vi "create instrument.vi"() -> ()   [LabVIEW 2020, in "Data.PG.lvclass"]
uses:
  Data.PG.lvclass
  <vilib>/numeric/Random Number (Range) U64.vi
  <vilib>/numeric/sub_Random U32.vi
  <vilib>/ErrorRing/Error Ring.xnode
panel:
  in  "Delete instrument":bool
  in  "Users":i32(listbox)
  out "new password":string
  out "new user name":string
  in  "path to object in table":string
  in  "new instrument password":string
  in  "Create instrument":bool
  in  "generate random password?":bool
  in  "new instrument name":string
  in  "STOP":bool
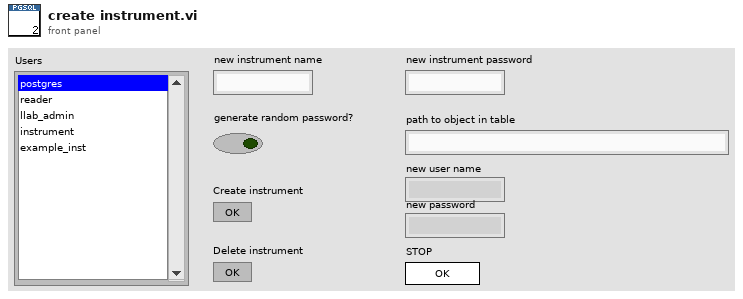
[diagram p1: front panel]
types:
  T1 = enum32{"Invalid", "Standard", "Closed", "Hidden", "Minimized", "Maximized"}
  T2 = enum32{"invalid app kind", "Development System", "Run Time System", "Student Edition", "Embedded LabVIEW", "Evaluation", "Custom"}
  T3 = cluster{"Core":cluster{"Current VI Reference":refnum<vi>, "Close Panel on Exit?":bool}, "connection info":cluster{"host":string, "port":string, "dbname":string, "user":string, "password":string}, "path to something in table":string, "new instrument name":string, "names already taken":string[], "Data.PG in":refnum<class "Data.PG.lvclass">, "Selected instrument":string, "Selected inst privileges":string[]}
  T4 = cluster{"host":string, "port":string, "dbname":string, "user":string, "password":string}
  T5 = cluster{"Current VI Reference":refnum<vi>, "Close Panel on Exit?":bool}
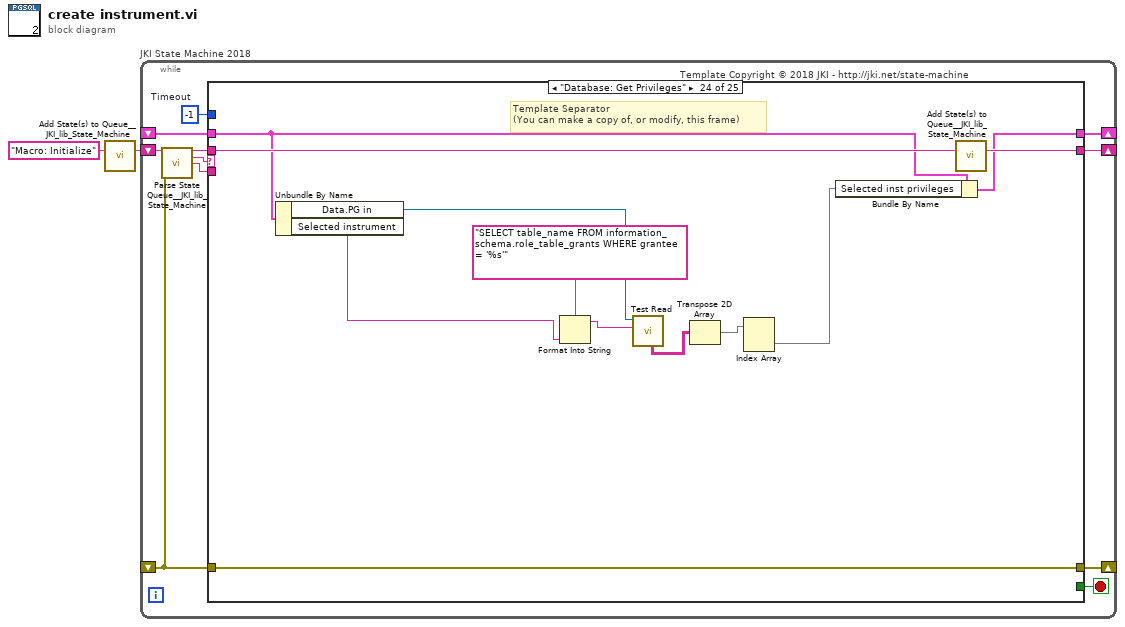
[diagram p0: block diagram]
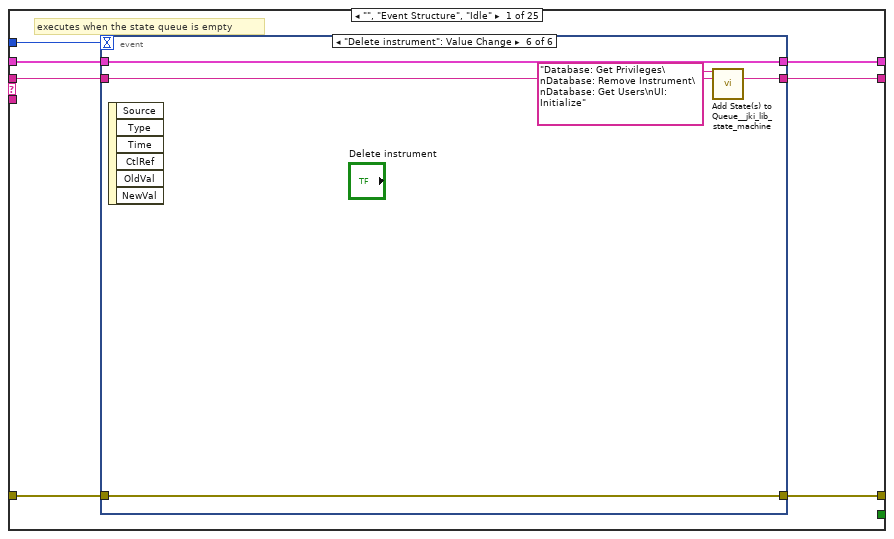
[diagram p2: hidden frame]
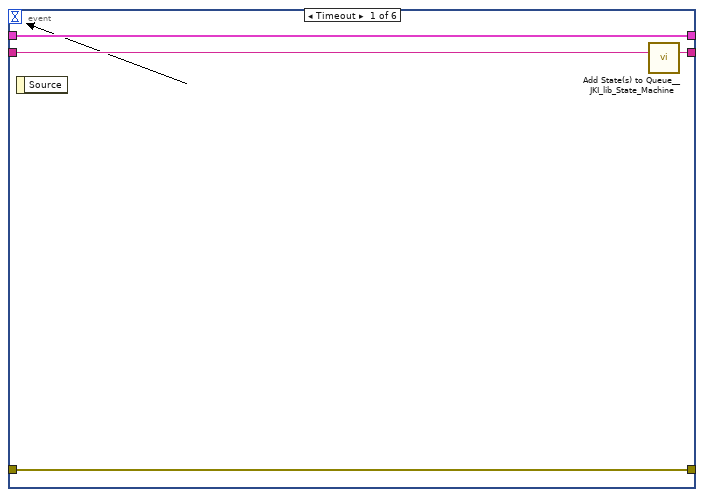
[diagram p3: hidden frame]
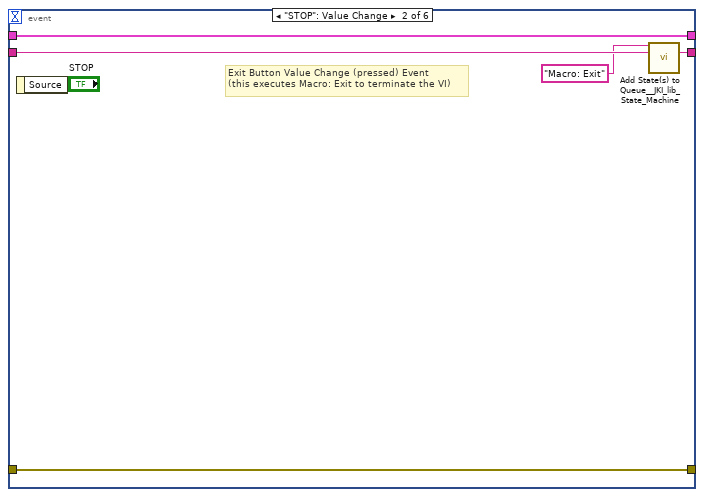
[diagram p4: hidden frame]
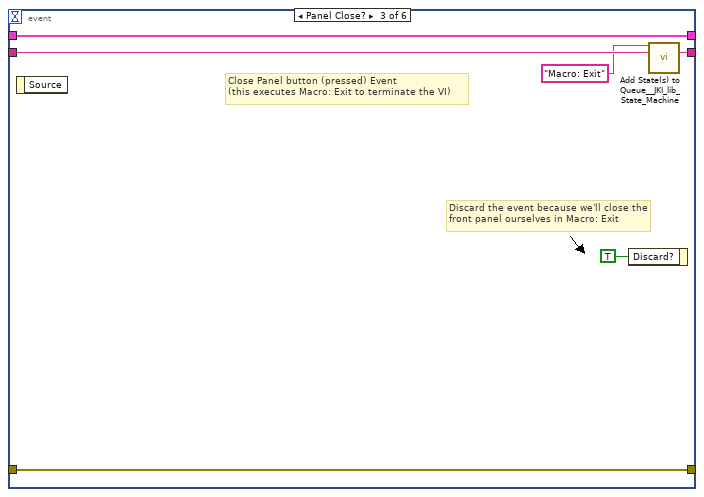
[diagram p5: hidden frame]
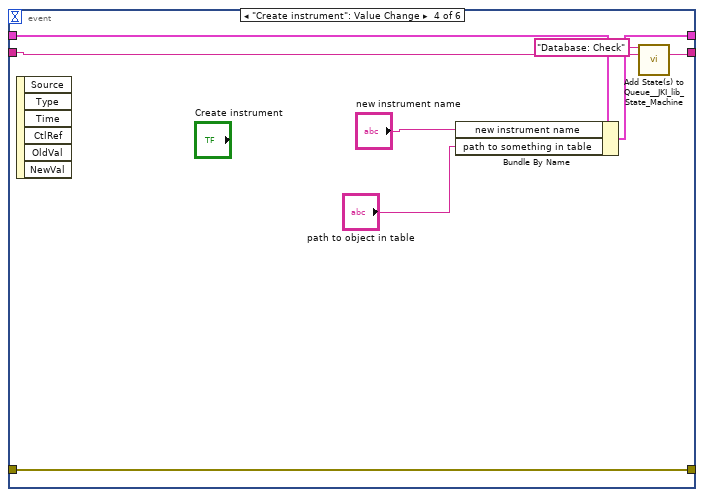
[diagram p6: hidden frame]
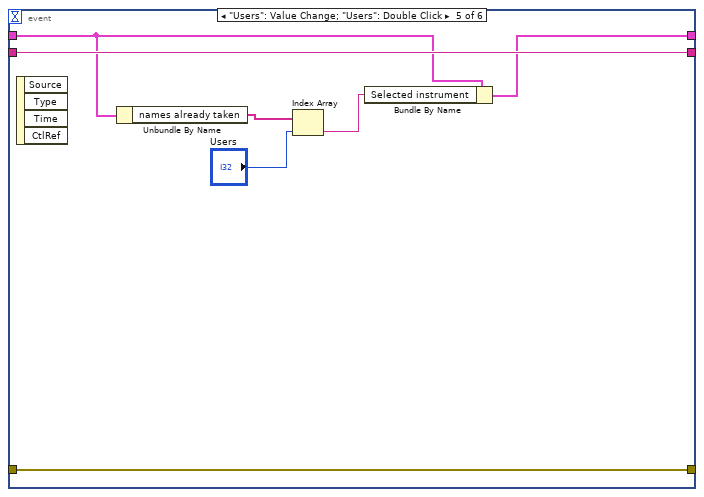
[diagram p7: hidden frame]
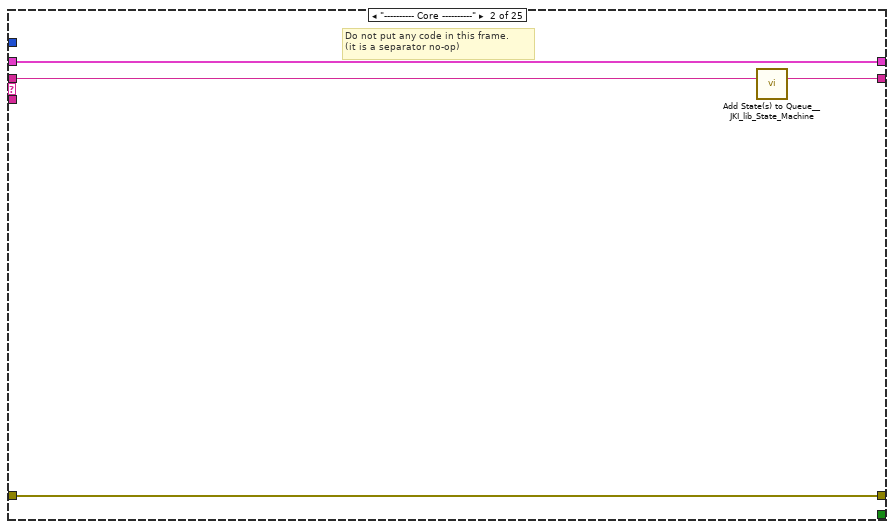
[diagram p8: hidden frame]
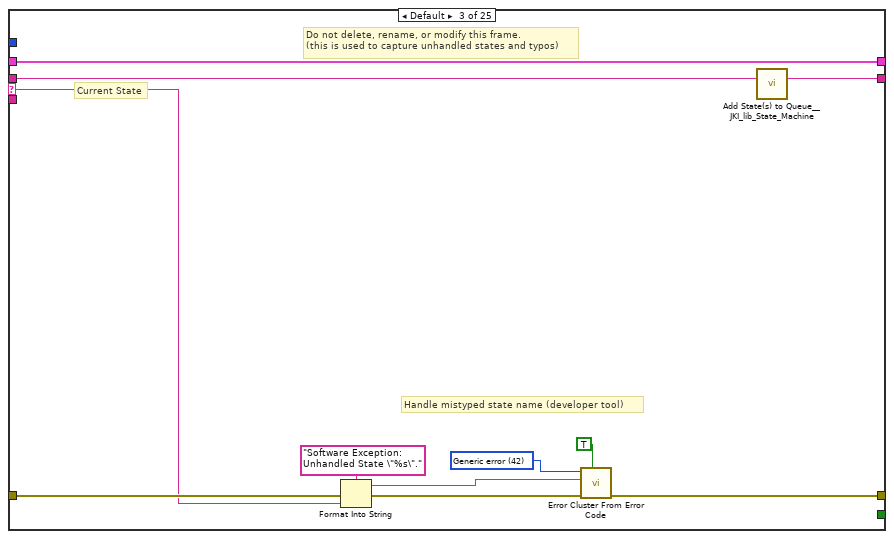
[diagram p9: hidden frame]
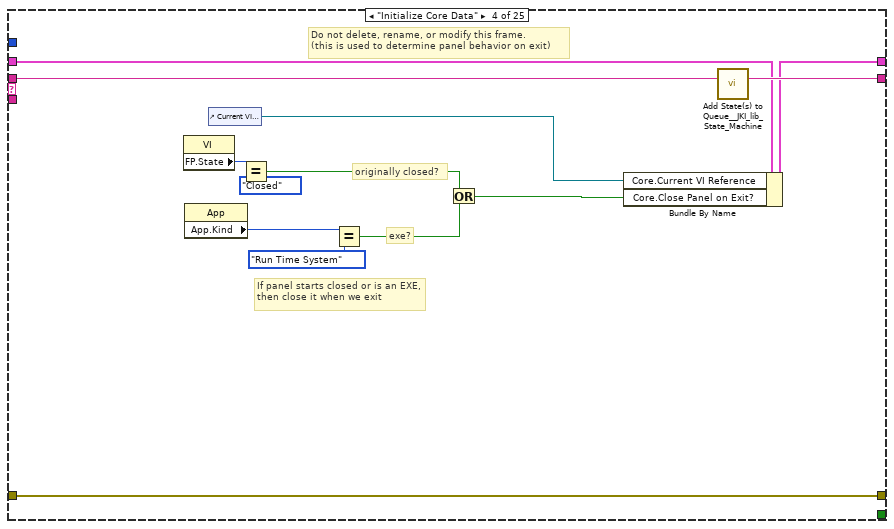
[diagram p10: hidden frame]
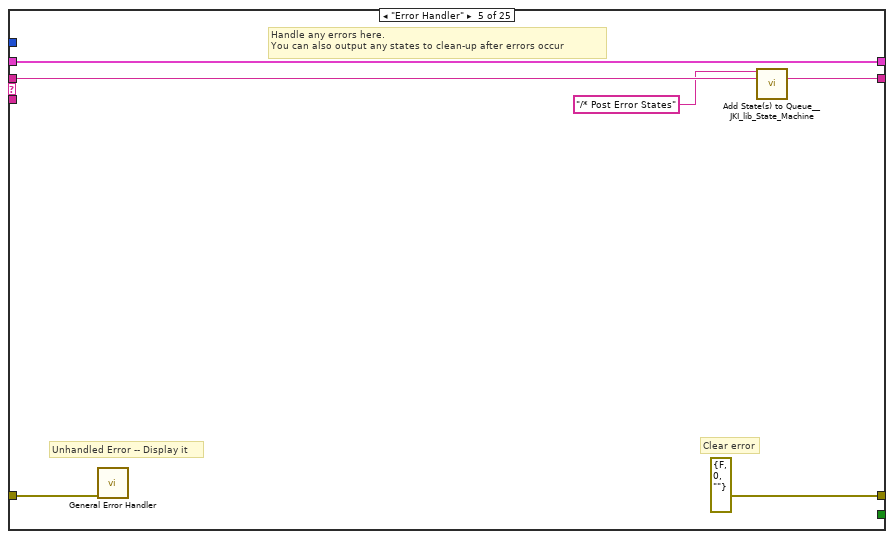
[diagram p11: hidden frame]
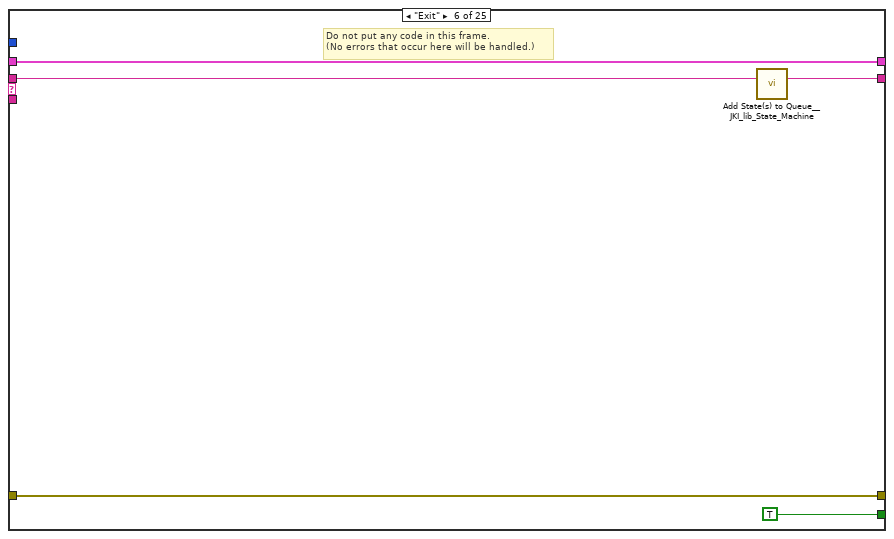
[diagram p12: hidden frame]
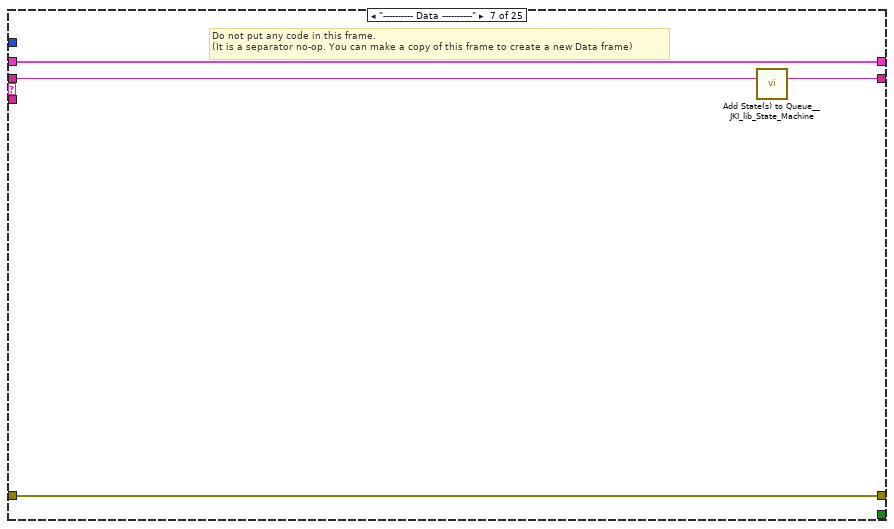
[diagram p13: hidden frame]
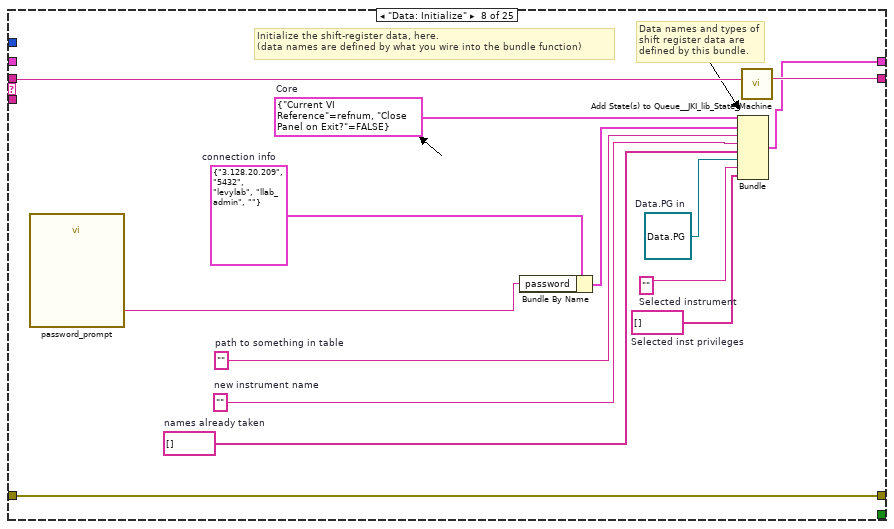
[diagram p14: hidden frame]
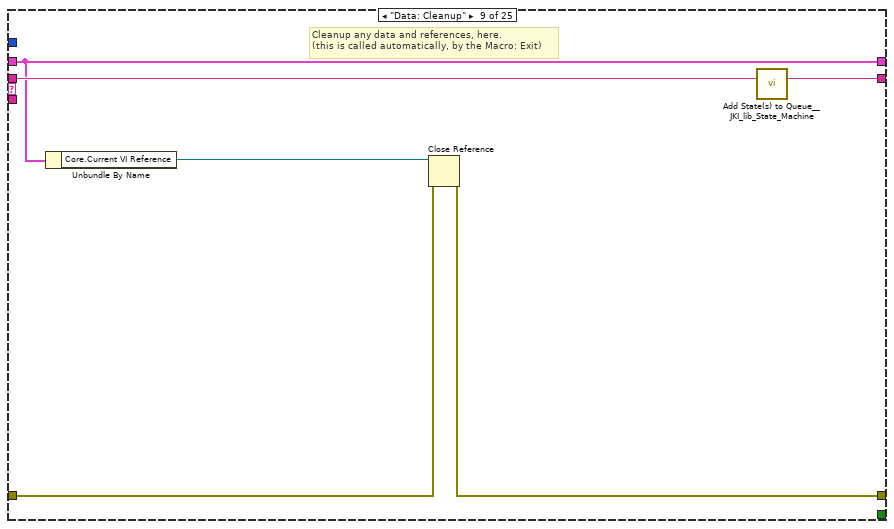
[diagram p15: hidden frame]
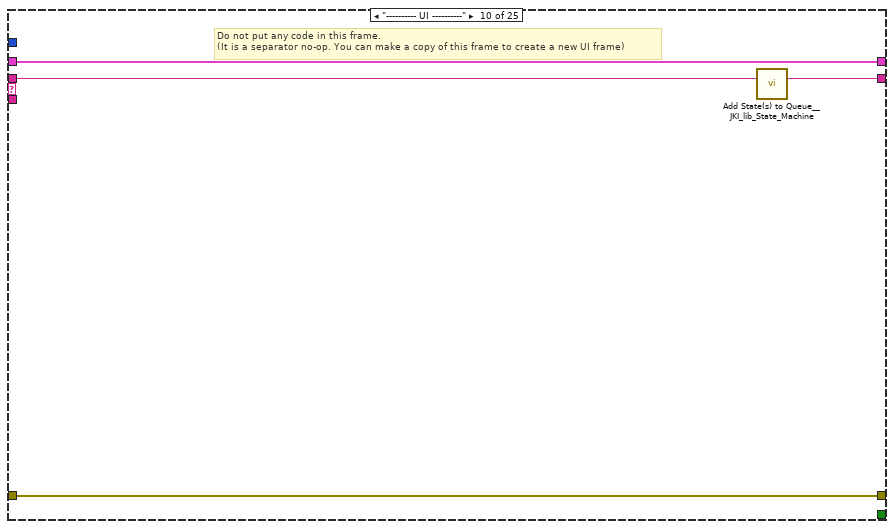
[diagram p16: hidden frame]
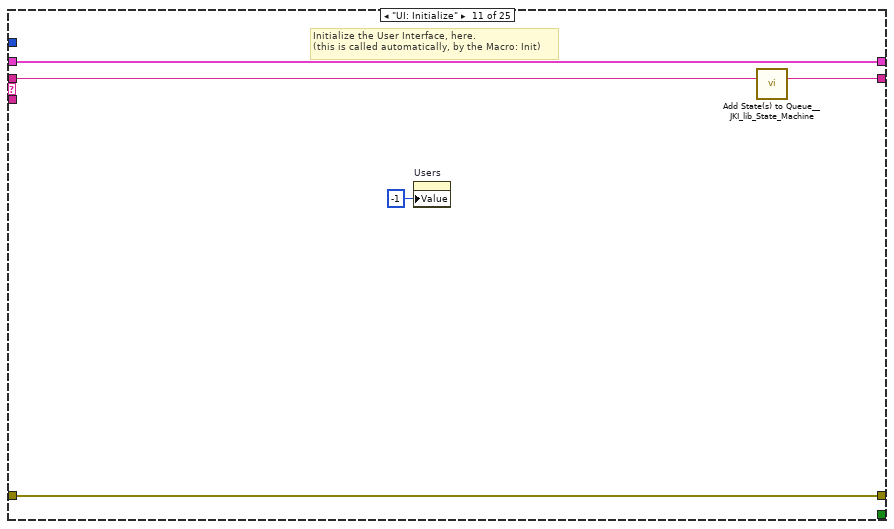
[diagram p17: hidden frame]
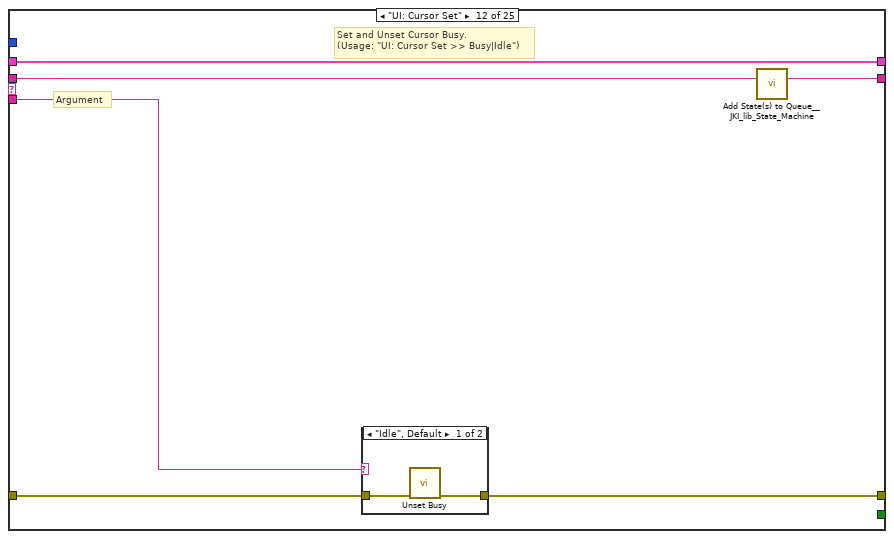
[diagram p18: hidden frame]
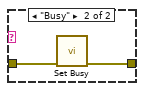
[diagram p19: hidden frame]
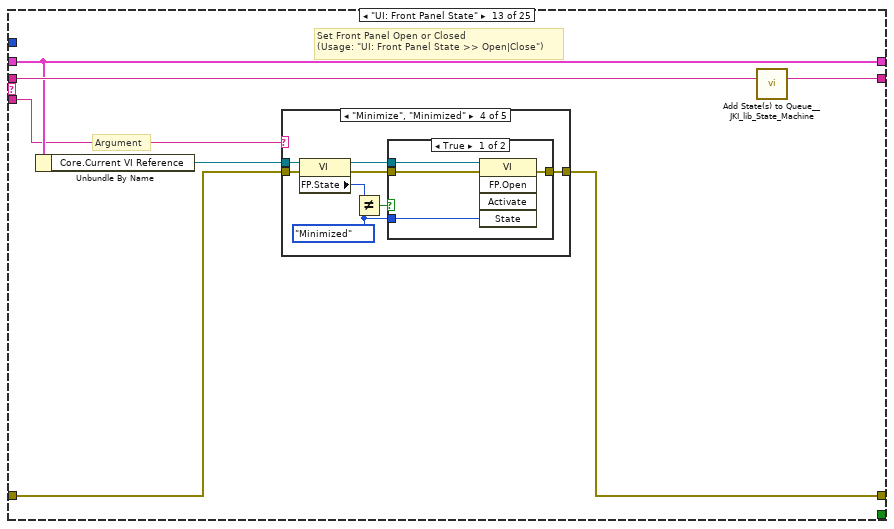
[diagram p20: hidden frame]
diagram:
  n1 = call <vilib>:"Add State(s) to Queue__JKI_lib_State_Machine.vi"("State(s) in (\"\")"="Macro: Initialize") -> ("States Out"=w2:string)  [unwired: 14 in]
  n2 = while "JKI State Machine 2018" {
    shift-right: [w6] -> _
    shift-left: _ -> [w5]
    shift-right: [w9] -> _
    shift-left: _ -> [w3]
    shift-right: [w8] -> _
    shift-left: w2 -> [w10]
    stop <- w7 stop-if-true
    w4 = -1  # Timeout
    # "Template Copyright © 2018 JKI - http://jki.net/state-machine"
    n3 = call <vilib>:"Parse State Queue__JKI_lib_State_Machine.vi"("State Queue"=w10, "Error In (no error)"=w3) -> ("Remaining States"=w12:string, "Current State"=w13:string, "Arguments"=w11:string)  [unwired: 11 in]
    n4 = case shown="\"Database: Get Privileges\"" w13 {
      selector: w13 -> [_ _ w60 _ _ _ _ _ _ _ _ _ _ _ _ _ _ _ _ _ _ _ _ _ _]
      tunnel: w12 -> [w20 w59 w64 w83 w89 w94 w98 w112 w118 w122 w127 w133 w144 w213 w218 w228 w232 w241 w247 w251 w262 w276 w313 w325 w334]
      tunnel: w11 -> [_ _ _ _ _ _ _ _ _ _ _ w128 w138 _ _ _ _ _ _ _ _ _ _ _ _]
      tunnel: w5 -> [w18 w56 w62 w76 w86 w92 w95 _ w113 w119 w125 w131 w140 w210 w215 w225 w229 w237 w243 w248 w254 w274 w308 w317 w332]
      tunnel: [w17 w57 w66 w80 errorcluster {"status"=FALSE, "code"=0, "source"=""} ("error out") w91 w96 w110 w114 w120 w124 w129 w141 w211 w216 w226 w230 w233 w244 w249 w256 w268 w309 w323 w331] -> w9
      tunnel: w3 -> [w16 w57 w65 w80 w85 w91 w96 w110 w115 w120 w124 w130 w142 w211 w216 w226 w230 w234 w245 w249 w257 w269 w310 w323 w326]
      tunnel: [w19 w58 w63 w82 w88 w93 w97 w111 w117 w121 w126 w132 w143 w212 w217 w227 w231 w240 w246 w250 w261 w275 w312 w324 w333] -> w8
      tunnel: [_ _ _ _ _ TRUE _ _ _ _ _ _ _ _ _ _ _ _ _ _ _ _ _ _ _] -> w7
      tunnel: [w15 w56 w62 w81 w86 w92 w95 w102 w113 w119 w125 w131 w140 w210 w215 w225 w229 w236 w243 w248 w253 w274 w308 w316 w332] -> w6
      tunnel: w4 -> [w14 _ _ _ _ _ _ _ _ _ _ _ _ _ _ _ _ _ _ _ _ _ _ _ _]
      frame "", "Event Structure", "Idle" {
        # "executes when the state queue is empty"
        n5 = event shown="[5] \"Delete instrument\": Value Change" {
          selector: _ -> [_ _ _ _ _ _]
          dyn-events: _ -> [_ _ _ _ _ _]
          timeout: w14 -> [_ _ _ _ _ _]
          tunnel: w20 -> [w24 w29 w35 w39 w49 w52]
          tunnel: [w23 w28 w34 w40 w49 w53] -> w19
          tunnel: w18 -> [w21 w26 w32 w43 w46 w54]
          tunnel: [w22 w27 w33 w38 w50 w55] -> w17
          tunnel: w16 -> [w22 w27 w33 w38 w50 w55]
          tunnel: [w21 w26 w32 w42 w45 w54] -> w15
          event Timeout {
            n6 = event-data() -> ()  [unwired: 1 in, 1 out]
            n7 = call <vilib>:"Add State(s) to Queue__JKI_lib_State_Machine.vi"("State(s) in (\"\")"=w24) -> ("States Out"=w23:string)  [unwired: 14 in]
          }
          event "STOP": Value Change {
            # "Exit Button Value Change (pressed) Event\n(this executes Macro: Exit to terminate the VI)"
            n8 = event-data() -> ()  [unwired: 1 in, 1 out]
            n9 = call <vilib>:"Add State(s) to Queue__JKI_lib_State_Machine.vi"("State(s) in Front (\"\")"="Macro: Exit", "State(s) in (\"\")"=w29) -> ("States Out"=w28:string)  [unwired: 13 in]
          }
          event Panel Close? {
            # "Discard the event because we'll close the front panel ourselves in Macro: Exit"
            # "Close Panel button (pressed) Event\n(this executes Macro: Exit to terminate the VI)"
            n10 = event-data() -> ()  [unwired: 1 in, 1 out]
            n11 = event-data("Discard?"=TRUE) -> ()  [unwired: 1 in, 1 out]
            n12 = call <vilib>:"Add State(s) to Queue__JKI_lib_State_Machine.vi"("State(s) in Front (\"\")"="Macro: Exit", "State(s) in (\"\")"=w35) -> ("States Out"=w34:string)  [unwired: 13 in]
          }
          event "Create instrument": Value Change {
            n13 = event-data() -> ()  [unwired: 1 in, 6 out]
            n14 = Bundle By Name(cluster=w43, "new instrument name"="new instrument name", "path to something in table"="path to object in table") -> (w42:T3)
            n15 = call <vilib>:"Add State(s) to Queue__JKI_lib_State_Machine.vi"("State(s) in Front (\"\")"="Database: Check" ("State(s) in Front (\"\")"), "State(s) in (\"\")"=w39) -> ("States Out"=w40:string)  [unwired: 13 in]
          }
          event "Users": Value Change; "Users": Double Click {
            n16 = event-data() -> ()  [unwired: 1 in, 4 out]
            n17 = Unbundle By Name(w46) -> ("names already taken"=w48:string[])
            n18 = Index Array(array=w48, index="Users") -> (element=w44:string)
            n19 = Bundle By Name(cluster=w46, "Selected instrument"=w44) -> (w45:T3)
          }
          event "Delete instrument": Value Change {
            n20 = event-data() -> ()  [unwired: 1 in, 6 out]
            n21 = call <vilib>:"Add State(s) to Queue__jki_lib_state_machine.vi"("State(s) in Front (\"\")"="Database: Get Privileges\nDatabase: Remove Instrument\nDatabase: Get Users\nUI: Initialize" ("State(s) in Front (\"\")"), "State(s) in (\"\")"=w52) -> ("States Out"=w53:string)  [unwired: 13 in]
          }
        }
      }
      frame "---------- Core ----------" {
        # "Do not put any code in this frame.\n(it is a separator no-op)"
        n22 = call <vilib>:"Add State(s) to Queue__JKI_lib_State_Machine.vi"("State(s) in (\"\")"=w59) -> ("States Out"=w58:string)  [unwired: 14 in]
      }
      frame Default {
        w69 = 42 items=["No error", "Argument error", "Memory is full", "Out of zone", "End of file", "File already open", "Generic file I/O error", "File not found", "File permission error", "Disk is full", "Duplicate path", "Too many files open", "System feature not enabled", "Resource file not found", "Cannot add resource", "Resource not found", "Image not found", "Image memory error", "Pen does not exist", "Config type invalid", "Config token not found", "Config parse error", "Config memory error", "Bad external code format", "Bad external code offset", "External code not present", "Null window", "Destroy window error", "Null menu", "Print aborted", "Bad print record", "Print driver error", "Windows error during printing", "Memory error during printing", "Print dialog error", "Generic print error", "Invalid device refnum", "Device not found", "Device parameter error", "Device unit error", "Cannot open device", "Device call aborted", "Generic error", "Cancelled by user", "Object ID too low", "Object ID too high", "Object not in heap", "Unknown heap", "Unknown object (invalid DefProc)", "Unknown object (DefProc not in table)", "Message out of range", "Invalid (null) method", "Unknown message", "Manager call not supported", "Bad address", "Network operation in progress", "Network operation timed out", "Connection is busy", "Network attribute not supported", "Network error", "Address in use", "System out of memory", "Connection aborted", "Connection refused", "Not connected", "Already connected", "Connection closed", "Initialization error (interapplication manager)", "Bad occurrence", "Wait on unbound occurrence handler", "Occurrence queue overflow", "Datalog type conflict", "Unused", "Unrecognized type (interapplication manager)", "Memory corrupt", "Failed to make temporary DLL", "Old CIN version", "Drag socket not found", "Failed to load drop-object", "Failed to register OLE object", "Failed to release OLE object", "Format specifier type mismatch", "Unknown format specifier", "Too few format specifiers", "Too many format specifiers", "Scan failed", "Newer CIN version", "Error converting to variant", "Runtime menu error", "Password tampered", "Variant attribute not found", "Incompatible variant data type", "Event data is not available", "Event Store is not present", "Occurrence is not found", "Event Queue is not created", "Event info is not available", "Refnum passed is NULL", "Error retrieving Class GUID", "Error retrieving CoClass GUID", "Error retrieving TypeLib GUID.", "Bad built application magic bytes.", "Specific driver is different from the specific driver associated with the Logical Name.", "There is no session opened to the class driver.", "Max Error", "MAX - Error with config objects", "MAX - Error loading configuration", "MAX - Group not supported"]
        # "Current State"
        # "Do not delete, rename, or modify this frame.\n(this is used to capture unhandled states and typos)"
        # "Handle mistyped state name (developer tool)"
        n23 = Format Into String(format string="Software Exception: Unhandled State \"%s\"." ("message"), error in=w65, w60) -> (resulting string=w68:string, error out=w67:errorcluster)  [unwired: 1 in]
        n24 = call <vilib>:"Error Cluster From Error Code.vi"("show call chain? (False)"=TRUE, "error in (no error)"=w67, "error message (\"\")"=w68, "error code (0)"=w69) -> ("error out"=w66:errorcluster)  [unwired: 5 in]
        n25 = call <vilib>:"Add State(s) to Queue__JKI_lib_State_Machine.vi"("State(s) in (\"\")"=w64) -> ("States Out"=w63:string)  [unwired: 14 in]
      }
      frame "Initialize Core Data" {
        # "Do not delete, rename, or modify this frame.\n(this is used to determine panel behavior on exit)"
        # "originally closed?"
        # "exe?"
        # "If panel starts closed or is an EXE, then close it when we exit"
        n26 = property class="VI"() -> ("FP.State"=w73:T1)  [unwired: 2 in, 2 out]
        n27 = property class="App"() -> ("App.Kind"=w79:T2)  [unwired: 2 in, 2 out]
        n28 = control-ref of="Current VI Reference"() -> (w74:refnum<vi>)
        n29 = Equal?(x=w73, y=T1."Closed" ("Front Panel Window:State")) -> (x = y?=w71:bool)
        n30 = Equal?(x=w79, y=T2."Run Time System" ("Application:Kind")) -> (x = y?=w77:bool)
        n31 = Or(x=w71, y=w77) -> (x .or. y?=w75:bool)
        n32 = Bundle By Name(cluster=w76, "Core.Current VI Reference"=w74, "Core.Close Panel on Exit?"=w75) -> (w81:T3)
        n33 = call <vilib>:"Add State(s) to Queue__JKI_lib_State_Machine.vi"("State(s) in (\"\")"=w83) -> ("States Out"=w82:string)  [unwired: 14 in]
      }
      frame "Error Handler" {
        # "Unhandled Error -- Display it"
        # "Handle any errors here.\nYou can also output any states to clean-up after errors occur"
        # "Clear error"
        n34 = call <vilib>:"General Error Handler.vi"("error in (no error)"=w85) -> ()  [unwired: 10 in, 5 out]
        n35 = call <vilib>:"Add State(s) to Queue__JKI_lib_State_Machine.vi"("State(s) in Front (\"\")"="/* Post Error States", "State(s) in (\"\")"=w89) -> ("States Out"=w88:string)  [unwired: 13 in]
      }
      frame "Exit" {
        # "Do not put any code in this frame.\n(No errors that occur here will be handled.)"
        n36 = call <vilib>:"Add State(s) to Queue__JKI_lib_State_Machine.vi"("State(s) in (\"\")"=w94) -> ("States Out"=w93:string)  [unwired: 14 in]
      }
      frame "---------- Data ----------" {
        # "Do not put any code in this frame.\n(It is a separator no-op. You can make a copy of this frame to create a new Data frame)"
        n37 = call <vilib>:"Add State(s) to Queue__JKI_lib_State_Machine.vi"("State(s) in (\"\")"=w98) -> ("States Out"=w97:string)  [unwired: 14 in]
      }
      frame "Data: Initialize" {
        w99 = string[] []  # Selected inst privileges
        w100 = ""  # Selected instrument
        w101 = refnum<class "Data.PG.lvclass"> refnum  # Data.PG in
        w104 = string[] []  # names already taken
        w105 = ""  # new instrument name
        w106 = ""  # path to something in table
        w109 = T4 {"host"="3.128.20.209", "port"="5432", "dbname"="levylab", "user"="llab_admin", "password"=""}  # connection info
        w103 = T5 {"Current VI Reference"=refnum, "Close Panel on Exit?"=FALSE}  # Core
        # "Data names and types of shift register data are defined by this bundle."
        # "Initialize the shift-register data, here.\n(data names are defined by what you wire into the bundle function)"
        n38 = call "password_prompt.vi"() -> ("password"=w107:string)  [unwired: 17 in, 2 out]
        n39 = Bundle By Name(cluster=w109, "password"=w107) -> (w108:T4)
        n40 = Bundle("Core"=w103, "connection info"=w108, "path to something in table"=w106, "new instrument name"=w105, "names already taken"=w104, "Data.PG in"=w101, "Selected instrument"=w100, "Selected inst privileges"=w99) -> (w102:T3)  [unwired: 1 in]
        n41 = call <vilib>:"Add State(s) to Queue__JKI_lib_State_Machine.vi"("State(s) in (\"\")"=w112) -> ("States Out"=w111:string)  [unwired: 14 in]
      }
      frame "Data: Cleanup" {
        # "Cleanup any data and references, here.\n(this is called automatically, by the Macro: Exit)"
        n42 = Unbundle By Name(w113) -> ("Core.Current VI Reference"=w116:refnum<vi>)
        n43 = Close Reference(reference=w116, error in (no error)=w115) -> (error out=w114:errorcluster)
        n44 = call <vilib>:"Add State(s) to Queue__JKI_lib_State_Machine.vi"("State(s) in (\"\")"=w118) -> ("States Out"=w117:string)  [unwired: 14 in]
      }
      frame "---------- UI ----------" {
        # "Do not put any code in this frame.\n(It is a separator no-op. You can make a copy of this frame to create a new UI frame)"
        n45 = call <vilib>:"Add State(s) to Queue__JKI_lib_State_Machine.vi"("State(s) in (\"\")"=w122) -> ("States Out"=w121:string)  [unwired: 14 in]
      }
      frame "UI: Initialize" {
        # "Initialize the User Interface, here.\n(this is called automatically, by the Macro: Init)"
        n46 = property on="Users" class="LstBox (strict)"("Value"=-1 ("Users")) -> ()  [unwired: 2 in, 2 out]
        n47 = call <vilib>:"Add State(s) to Queue__JKI_lib_State_Machine.vi"("State(s) in (\"\")"=w127) -> ("States Out"=w126:string)  [unwired: 14 in]
      }
      frame "UI: Cursor Set" {
        # "Argument"
        # "Set and Unset Cursor Busy.\n(Usage: \"UI: Cursor Set >> Busy|Idle\")"
        n48 = case shown="\"Idle\", Default" w128 {
          tunnel: w130 -> [w135 w137]
          tunnel: [w134 w136] -> w129
          frame "Idle", Default {
            n49 = call <vilib>:"Unset Busy.vi"("error in (no error)"=w135) -> ("error out"=w134:errorcluster)  [unwired: 10 in]
          }
          frame "Busy" {
            n50 = call <vilib>:"Set Busy.vi"("error in (no error)"=w137) -> ("error out"=w136:errorcluster)  [unwired: 9 in, 1 out]
          }
        }
        n51 = call <vilib>:"Add State(s) to Queue__JKI_lib_State_Machine.vi"("State(s) in (\"\")"=w133) -> ("States Out"=w132:string)  [unwired: 14 in]
      }
      frame "UI: Front Panel State" {
        # "Argument"
        # "Set Front Panel Open or Closed\n(Usage: \"UI: Front Panel State >> Open|Close\")"
        n52 = Unbundle By Name(w140) -> ("Core.Current VI Reference"=w139:refnum<vi>)
        n53 = case shown="\"Minimize\", \"Minimized\"" w138 {
          tunnel: w142 -> [w150 w165 w176 w189 w202]
          tunnel: [w152 w166 w178 w191 w204] -> w141
          tunnel: w139 -> [w151 w163 w177 w190 w203]
          frame "Open", "Standard", Default {
            w145 = T1."Standard" ("State")
            n54 = property class="VI"(reference=w151, error in=w150) -> (reference out=w148:refnum<vi>, error out=w149:errorcluster, "FP.State"=w147:T1)
            n55 = Not Equal?(x=w147, y=w145) -> (x != y?=w146:bool)
            n56 = case shown="True" w146 {
              tunnel: [w156 w158] -> w152
              tunnel: w149 -> [w155 w158]
              tunnel: w148 -> [w154 _]
              tunnel: w145 -> [w153 _]
              frame True {
                n57 = invoke class="VI" method="FP.Open"(reference=w154, error in=w155, "Activate"=TRUE, "State"=w153) -> (error out=w156:errorcluster)  [unwired: 1 in, 4 out]
              }
              frame False {
              }
            }
          }
          frame "Close", "Closed" {
            n58 = property class="VI"(reference=w163, error in=w165) -> (reference out=w162:refnum<vi>, error out=w164:errorcluster, "FP.State"=w160:T1)
            n59 = Not Equal?(x=w160, y=T1."Closed" ("Front Panel Window:State")) -> (x != y?=w159:bool)
            n60 = case shown="True" w159 {
              tunnel: [w167 w170] -> w166
              tunnel: w164 -> [w167 w169]
              tunnel: w162 -> [_ w168]
              frame False {
              }
              frame True {
                n61 = invoke class="VI" method="FP.Close"(reference=w168, error in=w169) -> (error out=w170:errorcluster)  [unwired: 1 in, 2 out]
              }
            }
          }
          frame "Hidden", "Hide" {
            w171 = T1."Hidden" ("State")
            n62 = property class="VI"(reference=w177, error in=w176) -> (reference out=w174:refnum<vi>, error out=w175:errorcluster, "FP.State"=w173:T1)
            n63 = Not Equal?(x=w173, y=w171) -> (x != y?=w172:bool)
            n64 = case shown="True" w172 {
              tunnel: [w182 w183] -> w178
              tunnel: w175 -> [w181 w183]
              tunnel: w174 -> [w180 _]
              tunnel: w171 -> [w179 _]
              frame True {
                n65 = invoke class="VI" method="FP.Open"(reference=w180, error in=w181, "State"=w179) -> (error out=w182:errorcluster)  [unwired: 2 in, 4 out]
              }
              frame False {
              }
            }
          }
          frame "Minimize", "Minimized" {
            w184 = T1."Minimized" ("State")
            n66 = property class="VI"(reference=w190, error in=w189) -> (reference out=w187:refnum<vi>, error out=w188:errorcluster, "FP.State"=w186:T1)
            n67 = Not Equal?(x=w186, y=w184) -> (x != y?=w185:bool)
            n68 = case shown="True" w185 {
              tunnel: [w195 w196] -> w191
              tunnel: w188 -> [w194 w196]
              tunnel: w187 -> [w193 _]
              tunnel: w184 -> [w192 _]
              frame True {
                n69 = invoke class="VI" method="FP.Open"(reference=w193, error in=w194, "State"=w192) -> (error out=w195:errorcluster)  [unwired: 2 in, 4 out]
              }
              frame False {
              }
            }
          }
          frame "Maximize", "Maximized" {
            w197 = T1."Maximized" ("State")
            n70 = property class="VI"(reference=w203, error in=w202) -> (reference out=w200:refnum<vi>, error out=w201:errorcluster, "FP.State"=w199:T1)
            n71 = Not Equal?(x=w199, y=w197) -> (x != y?=w198:bool)
            n72 = case shown="True" w198 {
              tunnel: [w208 w209] -> w204
              tunnel: w201 -> [w207 w209]
              tunnel: w200 -> [w206 _]
              tunnel: w197 -> [w205 _]
              frame True {
                n73 = invoke class="VI" method="FP.Open"(reference=w206, error in=w207, "State"=w205) -> (error out=w208:errorcluster)  [unwired: 2 in, 4 out]
              }
              frame False {
              }
            }
          }
        }
        n74 = call <vilib>:"Add State(s) to Queue__JKI_lib_State_Machine.vi"("State(s) in (\"\")"=w144) -> ("States Out"=w143:string)  [unwired: 14 in]
      }
      frame "---------- Macro ----------" {
        # "Do not put any code in this frame.\n(It is a separator no-op. You can make a copy of this frame to create a new Macro frame)"
        n75 = call <vilib>:"Add State(s) to Queue__JKI_lib_State_Machine.vi"("State(s) in (\"\")"=w213) -> ("States Out"=w212:string)  [unwired: 14 in]
      }
      frame "Macro: Initialize" {
        w214 = "Data: Initialize\nInitialize Core Data\nUI: Initialize\nUI: Front Panel State >> Open\nConnection: Open\nDatabase: Get Users"  # Data: Initialize Initialize Core Data UI: Initialize UI: Front Panel State >> Open Connection: Open Database: Get Users
        # "Initialization Macro\n(This is called once, when the VI starts)"
        n76 = call <vilib>:"Add State(s) to Queue__JKI_lib_State_Machine.vi"("State(s) in Front (\"\")"=w214, "State(s) in (\"\")"=w218) -> ("States Out"=w217:string)  [unwired: 13 in]
      }
      frame "Macro: Exit" {
        # "Exit Macro\n(This is called once, when the VI exits)"
        n77 = Unbundle By Name(w225) -> ("Core.Close Panel on Exit?"=w224:bool)
        n78 = Select(t="UI: Front Panel State >> Close", s=w224, f="") -> (s? t:f=w221:string)
        n79 = call <vilib>:"Add State(s) to Queue__JKI_lib_State_Machine.vi"("State(s) in (\"\")"=w221, "State(s) at Back (\"\")"="Data: Cleanup\nConnection: Close\nExit") -> ("States Out"=w219:string)  [unwired: 13 in]
        n80 = call <vilib>:"Add State(s) to Queue__JKI_lib_State_Machine.vi"("State(s) in Front (\"\")"=w219, "State(s) in (\"\")"=w228) -> ("States Out"=w227:string)  [unwired: 13 in]
      }
      frame "---------- Connection ----------" {
        # "Template Separator\n(You can make a copy of, or modify, this frame)"
        n81 = call <vilib>:"Add State(s) to Queue__JKI_lib_State_Machine.vi"("State(s) in (\"\")"=w232) -> ("States Out"=w231:string)  [unwired: 14 in]
      }
      frame "Connection: Open" {
        # "Your code here.\n(You can make a copy of, or modify, this frame)"
        n82 = Unbundle By Name(w237) -> ("Data.PG in"=w239:refnum<class "Data.PG.lvclass">, "connection info"=w238:T4)
        n83 = call "Set Connection Info.vi"("error in (no error)"=w234, "connection info"=w238, "Data.PG in"=w239) -> ("error out"=w233:errorcluster, "Data.PG out"=w235:refnum<class "Data.PG.lvclass">)  [unwired: 7 in]
        n84 = Bundle By Name(cluster=w237, "Data.PG in"=w235) -> (w236:T3)
        n85 = call <vilib>:"Add State(s) to Queue__JKI_lib_State_Machine.vi"("State(s) in (\"\")"=w241) -> ("States Out"=w240:string)  [unwired: 14 in]
      }
      frame "Connection: Close" {
        # "Your code here.\n(You can make a copy of, or modify, this frame)"
        n86 = Unbundle By Name(w243) -> ("Data.PG in"=w242:refnum<class "Data.PG.lvclass">)
        n87 = call-dynamic "Close.vi"("error in (no error)"=w245, "Data.PG in"=w242) -> ("error out"=w244:errorcluster)  [unwired: 8 in, 1 out]
        n88 = call <vilib>:"Add State(s) to Queue__JKI_lib_State_Machine.vi"("State(s) in (\"\")"=w247) -> ("States Out"=w246:string)  [unwired: 14 in]
      }
      frame "---------- Database ----------" {
        # "Template Separator\n(You can make a copy of, or modify, this frame)"
        n89 = call <vilib>:"Add State(s) to Queue__JKI_lib_State_Machine.vi"("State(s) in (\"\")"=w251) -> ("States Out"=w250:string)  [unwired: 14 in]
      }
      frame "Database: Get Users" {
        # "Template Separator\n(You can make a copy of, or modify, this frame)"
        n90 = Unbundle By Name(w254) -> ("Data.PG in"=w260:refnum<class "Data.PG.lvclass">)
        n91 = call-dynamic "Test Read.vi"("error in (no error)"=w257, "command"="SELECT usename FROM pg_catalog.pg_user;", "Data.PG in"=w260) -> ("error out"=w256:errorcluster, "Result"=w258:string[][])  [unwired: 3 in, 4 out]
        n92 = Transpose 2D Array(2D array=w258) -> (transposed array=w259:string[][])
        n93 = Index Array(array=w259) -> (element=w252:string[])  [unwired: 2 in]
        n94 = Bundle By Name(cluster=w254, "names already taken"=w252) -> (w253:T3)
        n95 = property on="Users" class="LstBox (strict)"("Item Names"=w252) -> ()  [unwired: 2 in, 2 out]
        n96 = call <vilib>:"Add State(s) to Queue__JKI_lib_State_Machine.vi"("State(s) in (\"\")"=w262) -> ("States Out"=w261:string)  [unwired: 14 in]
      }
      frame "Database: Check" {
        # "Template Separator\n(You can make a copy of, or modify, this frame)"
        n97 = Unbundle By Name(w274) -> ("names already taken"=w273:string[], "new instrument name"=w266:string)
        n98 = call <userlib>:"Search or Split String__ogtk.vi"("search string/char (-)"=" ", "string"=w266) -> ("offset after match"=w264:i32)  [unwired: 1 in, 2 out]
        n99 = Increment(x=w264) -> (x+1=w263:i32)
        n100 = for {
          tunnel: w273 -> [w292] mode=indexing
          tunnel: w266 -> [w291]
          shift-right: [w288] -> w272
          shift-left: w263 -> [w287]
          n101 = Equal?(x=w292, y=w291) -> (x = y?=w290:bool)
          n102 = case shown="False" w290 {
            tunnel: [0 1] -> w289
            frame False {
            }
            frame True {
            }
          }
          n103 = Add(x=w289, y=w287) -> (x+y=w288:i32)
        }
        n104 = Equal To 0?(x=w272) -> (x = 0?=w271:bool)
        n105 = case shown="False" w271 {
          tunnel: ["" "Database: Create User"] -> w270
          tunnel: [w277 w284] -> w267
          frame False {
            n106 = xnode "Error Ring"() -> ("error out"=w277:errorcluster)
          }
          frame True {
            n107 = xnode "Error Ring"() -> ("error out"=w284:errorcluster)
          }
        }
        n108 = Merge Errors(w267, w269) -> (w268:errorcluster)
        n109 = call <vilib>:"Add State(s) to Queue__jki_lib_state_machine.vi"("State(s) in Front (\"\")"=w270, "State(s) in (\"\")"=w276) -> ("States Out"=w275:string)  [unwired: 13 in]
      }
      frame "Database: Create User" {
        # "Template Separator\n(You can make a copy of, or modify, this frame)"
        n110 = Unbundle By Name(w308) -> ("Data.PG in"=w311:refnum<class "Data.PG.lvclass">, "new instrument name"=w296:string, "path to something in table"=w299:string)
        "new user name" <- w296
        n111 = call-poly <vilib>:"Random Number (Range).vi"("upper bound (100)"=u64 10000000000) -> ("number"=w303:u64)  [unwired: 10 in]
        n112 = Number To Decimal String(number=w303) -> (decimal integer string=w302:string)  [unwired: 1 in]
        n113 = Select(t=w302, s="generate random password?", f="new instrument password") -> (s? t:f=w300:string)
        "new password" <- w300
        n114 = Search/Split String(string=w299, search string/char (-)=":") -> (substring before match=w297:string)  [unwired: 1 in, 2 out]
        n115 = Format Into String(format string="CREATE ROLE %s login password '%s';\nGRANT INSERT ON %s TO %s;\nGRANT instrument to %s", w296, w300, w297, w296, w296) -> (resulting string=w307:string)  [unwired: 2 in, 1 out]
        n116 = call-dynamic "Test Read.vi"("error in (no error)"=w310, "command"=w307, "Data.PG in"=w311) -> ("error out"=w309:errorcluster)  [unwired: 3 in, 5 out]
        n117 = call <vilib>:"Add State(s) to Queue__JKI_lib_State_Machine.vi"("State(s) in Front (\"\")"="Database: Get Users" ("State(s) in Front (\"\")"), "State(s) in (\"\")"=w313) -> ("States Out"=w312:string)  [unwired: 13 in]
      }
      frame "Database: Get Privileges" {
        # "Template Separator\n(You can make a copy of, or modify, this frame)"
        n118 = Unbundle By Name(w317) -> ("Data.PG in"=w322:refnum<class "Data.PG.lvclass">, "Selected instrument"=w320:string)
        n119 = Format Into String(format string="SELECT table_name FROM information_schema.role_table_grants WHERE grantee = '%s'", w320) -> (resulting string=w314:string)  [unwired: 2 in, 1 out]
        n120 = call-dynamic "Test Read.vi"("command"=w314, "Data.PG in"=w322) -> ("Result"=w319:string[][])  [unwired: 4 in, 5 out]
        n121 = Transpose 2D Array(2D array=w319) -> (transposed array=w318:string[][])
        n122 = Index Array(array=w318) -> (element=w315:string[])  [unwired: 2 in]
        n123 = Bundle By Name(cluster=w317, "Selected inst privileges"=w315) -> (w316:T3)
        n124 = call <vilib>:"Add State(s) to Queue__JKI_lib_State_Machine.vi"("State(s) in (\"\")"=w325) -> ("States Out"=w324:string)  [unwired: 14 in]
      }
      frame "Database: Remove Instrument" {
        # "Template Separator\n(You can make a copy of, or modify, this frame)"
        n125 = Unbundle By Name(w332) -> ("Data.PG in"=w329:refnum<class "Data.PG.lvclass">, "Selected inst privileges"=w328:string[], "Selected instrument"=w327:string)
        n126 = case shown="\"False\", Default" w327 {
          tunnel: [w335 w352] -> w330
          tunnel: w329 -> [w343 _]
          tunnel: w328 -> [w342 _]
          tunnel: w327 -> [w338 _]
          tunnel: w326 -> [w337 _]
          frame "False", Default {
            n127 = for {
              tunnel: w343 -> [w351]
              shift-right: [w350] -> w341
              shift-left: _ -> [_]
              tunnel: w342 -> [w347] mode=indexing
              tunnel: w338 -> [w346]
              tunnel: w337 -> [w345]
              shift-right: [w344] -> w336
              shift-left: _ -> [_]
              n128 = Format Into String(format string="REVOKE INSERT ON %s FROM %s;", w347, w346) -> (resulting string=w349:string)  [unwired: 2 in, 1 out]
              n129 = call-dynamic "Test Read.vi"("error in (no error)"=w345, "command"=w349, "Data.PG in"=w351) -> ("error out"=w344:errorcluster, "Data.PG out"=w350:refnum<class "Data.PG.lvclass">)  [unwired: 3 in, 4 out]
            }
            n130 = Format Into String(format string="REVOKE instrument FROM %s;\nDROP ROLE %s;", w338, w338) -> (resulting string=w340:string)  [unwired: 2 in, 1 out]
            n131 = call-dynamic "Test Read.vi"("error in (no error)"=w336, "command"=w340, "Data.PG in"=w341) -> ("error out"=w335:errorcluster)  [unwired: 3 in, 5 out]
          }
          frame "instrument", "llab_admin", "postgres", "reader" {
            n132 = xnode "Error Ring"() -> ("error out"=w352:errorcluster)
          }
        }
        n133 = call <vilib>:"Add State(s) to Queue__JKI_lib_State_Machine.vi"("State(s) in (\"\")"=w334) -> ("States Out"=w333:string)  [unwired: 14 in]
        n134 = Merge Errors(w330, w326) -> (w331:errorcluster)
      }
    }
  }
